vi "buzzerTest.vi"() -> ()   [LabVIEW 2020]
uses:
  <vilib>/CISH Robotics/L4VMX VMXpi/Type Def/VMX Channel Index.ctl
  <vilib>/CISH Robotics/L4VMX VMXpi/Digital Output/Digital Output.lvclass
  <vilib>/CISH Robotics/L4VMX VMXpi/L4VMX.lvlib
panel:
  in  "BuzzerOn":bool
  in  "Stop Button":bool
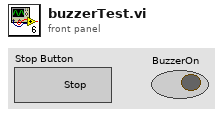
[diagram p1: front panel]
types:
  T1 = typedef "L4VMX.lvlib/VMX Channel Index.ctl" = enum16{"0", "1", "2", "3", "4", "5", "6", "7", "8", "9", "10", "11", "12", "13", "14", "15", "16", "17", "18", "19", "20", "21", "22", "23", "24", "25", "26", "27", "28", "29", "30", "31", "32", "33"}
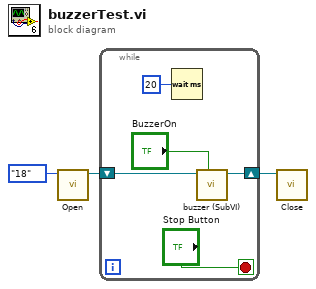
[diagram p0: block diagram]
diagram:
  n1 = call <vilib>:"Open.vi"("VMX Channel Index"=VMX_Channel_Index."18") -> ("Digital Output Object"=w3:refnum<class "Digital Output.lvclass">)  [unwired: 9 in, 1 out]
  n2 = while {
    shift-right: [w7] -> w2
    shift-left: w3 -> [w8]
    stop <- "Stop Button" stop-if-true
    n3 = Wait (ms)(milliseconds to wait=u32 20) -> ()  [unwired: 1 out]
    n4 = call "buzzer (SubVI).vi"("BuzzerOn"="BuzzerOn", "Digital Output in"=w8) -> ("Digital Output out"=w7:refnum<class "Digital Output.lvclass">)  [unwired: 8 in, 1 out]
  }
  n5 = call <vilib>:"Close.vi"("Digital Output Object"=w2) -> ()  [unwired: 10 in, 1 out]
